vi "Select Channel.vi"(8 "error in (no error)":errorcluster, 10 "Channel":i32, 11 "LakeShore 370 Driver in":refnum<class "LakeShore 370 Driver.lvclass">) -> (0 "error out":errorcluster, 3 "LakeShore 370 Driver out":refnum<class "LakeShore 370 Driver.lvclass">)   [LabVIEW 2024, in "LakeShore 370 Driver.lvclass"]
uses:
  LakeShore 370 Driver.lvclass
  LakeShore 370 Driver.lvclass/LakeShore 370 Driver.ctl
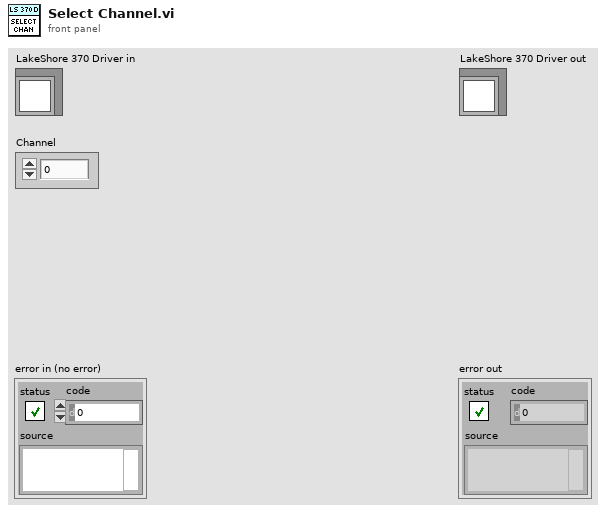
[diagram p1: front panel]
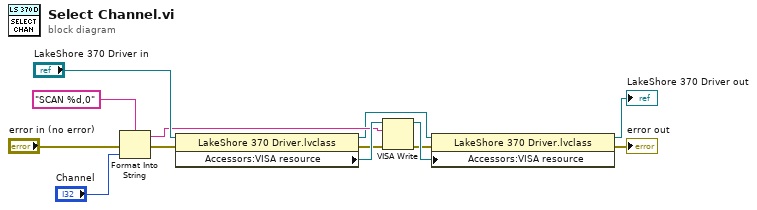
[diagram p0: block diagram]
diagram:
  n1 = Format Into String(format string="SCAN %d,0", error in="error in (no error)", "Channel") -> (resulting string=w6:string, error out=w8:errorcluster)  [unwired: 1 in]
  n2 = property class="LakeShore 370 Driver.lvclass"(reference="LakeShore 370 Driver in", error in=w8) -> (reference out=w5:refnum<class "LakeShore 370 Driver.lvclass">, error out=w7:errorcluster, "Accessors:VISA resource"=w9:refnum<visa-resource-name>)
  n3 = VISA Write(VISA resource name=w9, write buffer=w6, error in (no error)=w7) -> (VISA resource name out=w4:refnum<visa-resource-name>, error out=w3:errorcluster)  [unwired: 1 out]
  n4 = property class="LakeShore 370 Driver.lvclass"(reference=w5, error in=w3, "Accessors:VISA resource"=w4) -> (reference out=→"LakeShore 370 Driver out":refnum<class "LakeShore 370 Driver.lvclass">, error out=→"error out":errorcluster)
